vi "MoveRelate.vi"(8 "error in (no error)":errorcluster, 11 "ZanClass in":refnum<class "ZanClass.lvclass">) -> (0 "error out":errorcluster, 3 "ZanClass out":refnum<class "ZanClass.lvclass">)   [LabVIEW 2019, in "ZanClass.lvclass"]
uses:
  ZanClass.lvclass
  LLB/zmotion/zaux/zauxdll.lvlib
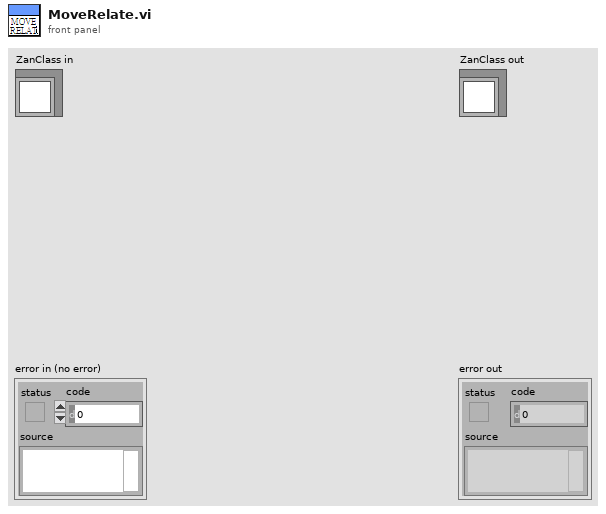
[diagram p1: front panel]
types:
  T1 = cluster{"AxisName":string, "Accel":dbl, "Deaccel":dbl, "Speed":dbl, "Sramp":dbl}[]
  T2 = typedef "IO Card_Type.ctl" = enum16{"None", "Unidaq32", "6480", "2410C-64", "Zan", "DMC1000B", "16InOut", "Robot", "DMC3600"}
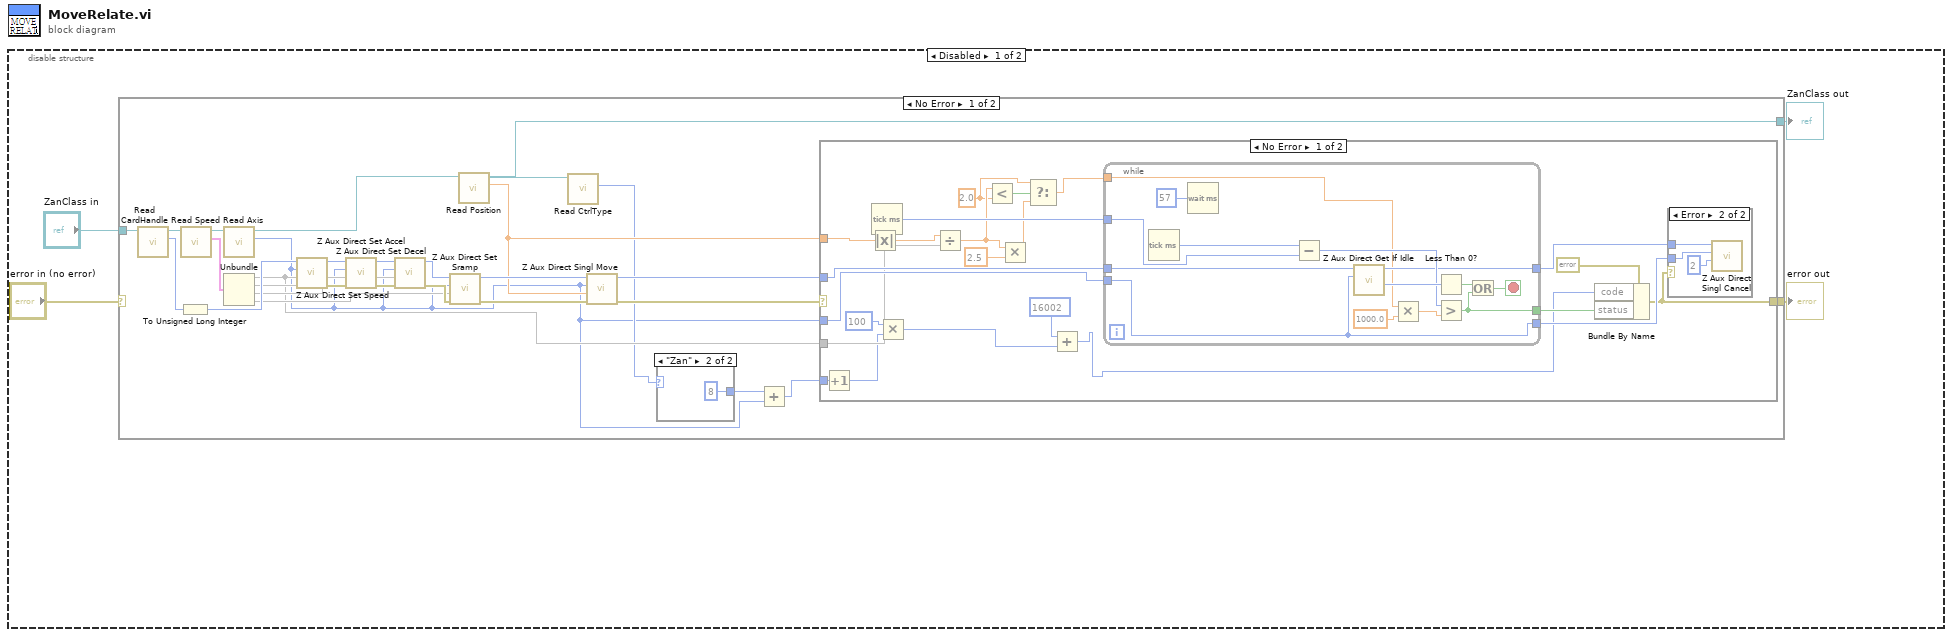
[diagram p0: block diagram]
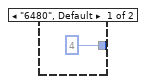
[diagram p2: hidden frame]
diagram:
  n1 = disable-structure shown="Disabled" {
    frame Disabled {
      n2 = case shown="No Error" "error in (no error)" {
        selector: "error in (no error)" -> [_ w76]
        tunnel: "ZanClass in" -> [w32 w77]
        tunnel: [w10 w76] -> w2
        tunnel: [w9 w77] -> w1
        frame No Error {
          n3 = call-dynamic "Read CardHandle.vi"("AxisCard in"=w32) -> ("CardHandle"=w31:i32, "AxisCard out"=w26:refnum<class "ZanClass.lvclass">)  [unwired: 8 in, 1 out]
          n4 = To Unsigned Long Integer(number=w31) -> (unsigned 32bit integer=w30:u32)
          n5 = call-dynamic "Read Speed.vi"("AxisCard in"=w26) -> ("AxisSpeed"=w24:T1, "AxisCard out"=w25:refnum<class "ZanClass.lvclass">)  [unwired: 8 in, 1 out]
          n6 = call-dynamic "Read Axis.vi"("AxisCard in"=w25) -> ("Axis"=w5:u32, "AxisCard out"=w16:refnum<class "ZanClass.lvclass">)  [unwired: 8 in, 1 out]
          n7 = Unbundle(w24) -> (w12, w23, w19, w18)
          n8 = call "Z Aux Direct Set Speed.vi"("fValue"=w12, "iaxis"=w5, "handle"=w30) -> ("error out"=w22:errorcluster, "handle out"=w29:u32)  [unwired: 6 in, 1 out]
          n9 = call "Z Aux Direct Set Accel.vi"("error in (no error)"=w22, "fValue"=w23, "iaxis"=w5, "handle"=w29) -> ("error out"=w21:errorcluster, "handle out"=w28:u32)  [unwired: 5 in, 1 out]
          n10 = call "Z Aux Direct Set Decel.vi"("error in (no error)"=w21, "fValue"=w19, "iaxis"=w5, "handle"=w28) -> ("error out"=w20:errorcluster, "handle out"=w27:u32)  [unwired: 5 in, 1 out]
          n11 = call "Z Aux Direct Set Sramp.vi"("error in (no error)"=w20, "fValue"=w18, "iaxis"=w5, "handle"=w27) -> ("error out"=w15:errorcluster, "handle out"=w17:u32)  [unwired: 5 in, 1 out]
          n12 = call-dynamic "Read Position.vi"("AxisCard in"=w16) -> ("Position"=w11:dbl, "AxisCard out"=w9:refnum<class "ZanClass.lvclass">)  [unwired: 8 in, 1 out]
          n13 = call-dynamic "Read CtrlType.vi"("AxisCard in"=w9) -> ("IO Card Type"=w8:T2)  [unwired: 8 in, 2 out]
          n14 = call "Z Aux Direct Singl Move.vi"("error in (no error)"=w15, "fdistance"=w11, "iaxis"=w5, "handle"=w17) -> ("error out"=w14:errorcluster, "handle out"=w13:u32)  [unwired: 5 in, 1 out]
          n15 = case shown="\"Zan\"" w8 {
            tunnel: [4 8] -> w7
            frame "6480", Default {
            }
            frame "Zan" {
            }
          }
          n16 = Add(x=w7, y=w5) -> (x+y=w6:u32)
          n17 = case shown="No Error" w14 {
            selector: w14 -> [_ w75]
            tunnel: w13 -> [w57 _]
            tunnel: w5 -> [w52 _]
            tunnel: w12 -> [w46 _]
            tunnel: w11 -> [w47 _]
            tunnel: [w49 w75] -> w10
            tunnel: w6 -> [w37 _]
            frame No Error {
              w41 = 2.0 ("y")
              n18 = Increment(x=w37) -> (x+1=w36:u32)
              n19 = Absolute Value(x=w47) -> (abs(x)=w40:dbl)
              n20 = Tick Count (ms)() -> (millisecond timer value=w56:u32)
              n21 = Multiply(x=u32 100, y=w36) -> (x*y=w35:u32)
              n22 = Divide(x=w40, y=w46) -> (x/y=w45:dbl)
              n23 = Less?(x=w45, y=w41) -> (x < y?=w44:bool)
              n24 = Multiply(x=w45, y=2.5) -> (x*y=w43:dbl)
              n25 = Select(t=w41, s=w44, f=w43) -> (s? t:f=w42:dbl)
              n26 = Add(x=16002, y=w35) -> (x+y=w39:u32)
              n27 = while {
                tunnel: w57 -> [w74]
                tunnel: w52 -> [w62]
                tunnel: w56 -> [w69]
                tunnel: [w64] -> w54
                tunnel: [w63] -> w51
                tunnel: [w62] -> w50
                tunnel: w42 -> [w61]
                stop <- w65 stop-if-true
                n28 = Tick Count (ms)() -> (millisecond timer value=w70:u32)
                n29 = Wait (ms)(milliseconds to wait=u32 57) -> ()  [unwired: 1 out]
                n30 = Subtract(x=w70, y=w69) -> (x-y=w68:u32)
                n31 = call "Z Aux Direct Get If Idle.vi"("iaxis"=w62, "handle"=w74) -> ("piValue out"=w73:i32, "handle out"=w63:u32)  [unwired: 6 in, 2 out]
                n32 = Multiply(x=w61, y=1000.0) -> (x*y=w67:dbl)
                n33 = Less Than 0?(x=w73) -> (x < 0?=w66:bool)
                n34 = Greater?(x=w68, y=w67) -> (0:w64:bool)
                n35 = Or(x=w66, y=w64) -> (x .or. y?=w65:bool)
              }
              n36 = Bundle By Name(cluster=errorcluster {"status"=FALSE, "code"=16601, "source"="MoveTimeOut"} ("error constant"), "code"=w39, "status"=w54) -> (w49:errorcluster)
              n37 = case shown="Error" w49 {
                tunnel: w51 -> [_ w60]
                tunnel: w50 -> [_ w59]
                frame No Error {
                }
                frame Error {
                  n38 = call "Z Aux Direct Singl Cancel.vi"("imode"=2, "iaxis"=w59, "handle"=w60) -> ()  [unwired: 6 in, 3 out]
                }
              }
            }
            frame Error {
            }
          }
        }
        frame Error {
        }
      }
      "error out" <- w2
      "ZanClass out" <- w1
    }
    frame Enabled {
    }
  }
